vi "Save_Source.vi"(8 "error in (no error)":errorcluster, 11 "AB_Build in":refnum<class "AB_Build.lvclass">) -> (0 "error out":errorcluster, 3 "AB_Build out":refnum<class "AB_Build.lvclass">)   [LabVIEW 2020, in "AB_Build.lvclass"]
uses:
  <vilib>/AppBuilder/AB_Classes/Build/AB_Build.lvclass
  <vilib>/AppBuilder/AB_Classes/Build/AB_Build.lvclass/AB_Build.ctl
  <vilib>/AppBuilder/AB_Classes/Source/AB_Source.lvclass
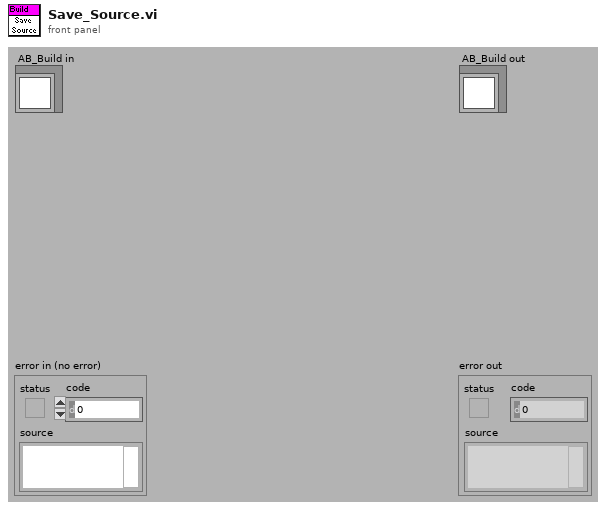
[diagram p1: front panel]
types:
  T1 = typedef "ItemRef.ctl" = u64
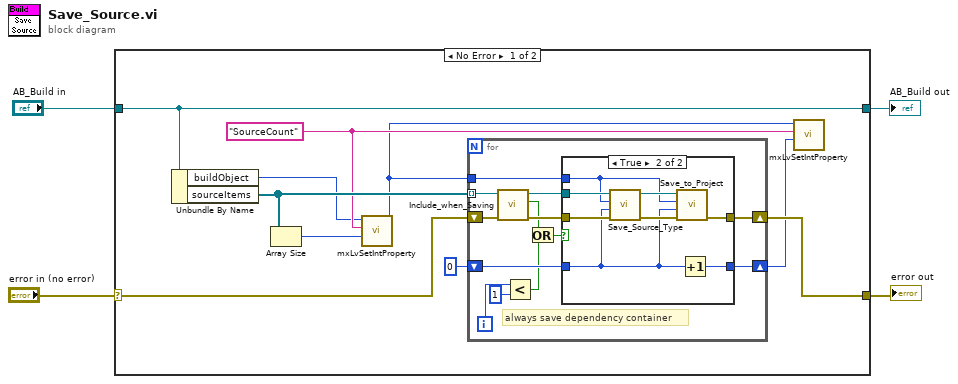
[diagram p0: block diagram]
diagram:
  n1 = case shown="No Error" "error in (no error)" {
    selector: "error in (no error)" -> [w11 w39]
    tunnel: [w10 w39] -> w3
    tunnel: [w14 w38] -> w1
    tunnel: "AB_Build in" -> [w14 w38]
    frame No Error {
      w7 = "SourceCount"
      n2 = Unbundle By Name(w14) -> ("buildObject"=w5:T1, "sourceItems"=w12:refnum<class "AB_Source.lvclass">[])
      n3 = Array Size(array=w12) -> (size(s)=w13:i32)
      n4 = call <resource>:"mxLvSetIntProperty.vi"("Value (0)"=w13, "Tag"=w7, "Item"=w5) -> ("Item"=w6:T1)  [unwired: 7 in, 1 out]
      n5 = for {
        tunnel: w12 -> [w25] mode=indexing
        tunnel: w6 -> [w27]
        shift-right: [w26] -> w10
        shift-left: w11 -> [w23]
        shift-right: [w20] -> w8
        shift-left: 0 -> [w21]
        i -> [w17]
        # "always save dependency container"
        n6 = call-dynamic "Include_when_Saving.vi"("error in (no error)"=w23, "AB_Source in"=w25) -> ("error out"=w22:errorcluster, "include"=w19:bool, "AB_Source out"=w24:refnum<class "AB_Source.lvclass">)  [unwired: 7 in]
        n7 = Less?(x=w17, y=1) -> (x < y?=w15:bool)
        n8 = Or(x=w19, y=w15) -> (x .or. y?=w18:bool)
        n9 = case shown="True" w18 {
          tunnel: w24 -> [_ w35]
          tunnel: w27 -> [_ w31]
          tunnel: [w29 w37] -> w26
          tunnel: w22 -> [w29 w33]
          tunnel: w21 -> [w28 w30]
          tunnel: [w28 w36] -> w20
          frame False {
          }
          frame True {
            n10 = call-dynamic "Save_Source_Type.vi"("error in (no error)"=w33, "index"=w30, "buildObject"=w31, "AB_Source in"=w35) -> ("error out"=w32:errorcluster, "AB_Source out"=w34:refnum<class "AB_Source.lvclass">)  [unwired: 6 in]
            n11 = call-dynamic "Save_to_Project.vi"("error in (no error)"=w32, "index"=w30, "buildObject"=w31, "AB_Source in"=w34) -> ("error out"=w37:errorcluster)  [unwired: 6 in, 1 out]
            n12 = Increment(x=w30) -> (x+1=w36:i32)
          }
        }
      }
      n13 = call <resource>:"mxLvSetIntProperty.vi"("Value (0)"=w8, "Tag"=w7, "Item"=w6) -> ()  [unwired: 7 in, 2 out]
    }
    frame Error {
    }
  }
  "error out" <- w3
  "AB_Build out" <- w1
